vi "Read Serial Number Folder.vi"(8 "error in":errorcluster, 11 "Data IN":T1={"Message"="", "Homed?"=FALSE, "NextState"=enum."Timeout", "G.Load"=0.0, "G.Position"=0.0, "Load#"=0, "[G.Loads]"=[], "[TotalLoads]"=[], "[Errors]"=[], "ZeroWait"=0, "Results"=[], "DwellWait"=FALSE, "Test Result"=FALSE, "[CondyleLoads]"=[], "[Max]"=[], "[Min]"=[], "Valid String?"=FALSE, "ScanTime"=timestamp(0 s since 1904-01-01), "ScannedString"="", "LabelDevID"=0, "MfgDate"=timestamp(0 s since 1904-01-01), "[EEPROM Cmds]"=[], "[CalData]"=[], "[A/Ds]"=[], "[A/Dmax]"=[], "[A/Dmin]"=[], "BattMax"=0.0, "BattMin"=0.0, "DwellTime"=2000, "PendingDeviceType"="", "Zero G.load"=0.0, "GAINC Value"="", "Programming Step"=enum."Load EEPROM", "Front Panel Program?"=FALSE, "Final Program?"=FALSE, "PCB Score"=100, "AssyScore"=100, "Pass/Fail #"="", "Result String"="", "Programming Mode"=enum."Initial Program", "Angle Test Step"=enum."Initialize", "Accel Values"=[], "Shutdown Counter"=0, "V1"=0, "V2"=0, "V3"=0, "V4"=0, "EEPROM Data"=[], "Counter"=0, "Page#"=0, "Timer"=timestamp(0 s since 1904-01-01), "Use Mark10?"=FALSE, "Eng-Result#"=0, "DUT Serial #"=0, "Scroll Message?"=FALSE, "Clear Message"=FALSE, "Batt Test Step "=enum."Initialize", "RXTX Window Found?"=FALSE, "Shutdown First Call?"=FALSE, "A2 Delay (msec)"=500, "Support Script"={"Script #"="", "Script Revision"="", "[OEMs]"=[], "[[DeviceTypes]]"=[], "[[DeviceTypesVals]]"=[], "[[List of Errors]]"=[], "Default GAINC"="", "[[ASICtrims]]"=[], "ID For Echo"="", "Condyle A CalFactor"=100, "Condyle B CalFactor"=100, "[OEMs Prefix]"=[], "Packet ID 18"="", "[[Force Table Load Test]]"=[], "[[Force Table AccurTest]]"=[]}, "Serial Table"={"Serial File Path"=path "", "[[Serial Lookup Table]]"=[], "Serial Device Info"=[], "Valid Serial?"=FALSE}, "Target Information"={"Target Brand"="", "Target DeviceType"="", "Target Serial#"=100, "Target Lot#"=0, "Target DevID"=0, "Target Channel"=5}, "Operator"="", "COM Port"="", "Config Path"=path "", "Tx Array"=[], "DUT Parameters"={"Channel"=0, "DeviceID"=0, "Script Rev"=0, "Month"=0, "Day"=0, "Year"=0, "Lot#"=0, "V1"=0, "V2"=0, "V3"=0, "V4"=0, "MFG"=0, "Cal FactorA 10"=0, "Cal FactorB 10  "=0, "Cal FactorA 16"=0, "Cal FactorB 16"=0, "ASICtrim"=[], "TmpChan"=0, "GAINC"="", "Brand"="", "Device"="", "Serial #"=0, "Batt310"=0, "Batt 280"=0}, "FTS Main?"=FALSE, "Loading"={"[Forces]"=[], "[Dwell]"=[], "Loading Step"=enum."Initialize Test"}, "Software Version"="", "Correction Factor"="", "Second Load Test"=FALSE, "Acc Loads"=[], "Mark10 Config"={"H2S%"=[80.0, 85.0, 90.0, 95.0, 100.0], "H2S Speed"=[12.0, 8.0, 6.0, 4.0, 2.0], "H to S"=2.0, "Home Speed"=1.0, "LoadWin"=0.0, "Load Speed"=0.0, "PID"={"Kp"=0.04, "Kd"=0.005001, "Ki"=2.9999999999999923e-05}}, "Channels"={"Transceiver Ch"=5, "Operating Ch"=5, "Start Ch"=0}, "Channel EEPROM"=[], "Load Notes"=[], "Engr Log?"=FALSE, "Time"=[], "Program Retry"=FALSE, "Operator Channel"="", "Target Channel "="", "New Data Program"=FALSE, "NFHU Pass?"=FALSE, "Cycle Number"=0, "Cal Cycle#"=0, "[Avg G.Loads] "=[], "[Avg A/Ds] "=[], "Cal Retry?"=FALSE, "[Total A/Ds]  "=[], "Cycle Num LA"=0, "LA Cycle# "=0, "Shim Num"=0, "Shim#  "=0, "Angle Test?"=FALSE} {"Mark10 Config"."PID"."Ki" min=0.0 max=200.0 format="%.6f"; "Mark10 Config"."PID"."Kd" min=0.0 max=200.0 format="%.6f"; "Mark10 Config"."PID"."Kp" min=0.0 max=200.0 format="%.6f"; "DUT Parameters"."ASICtrim" format="%02x"}) -> (0 "error out":errorcluster, 2 "Current State Out":T2=enum."Scan Channels", 3 "State-machine Local Variables out":T1={"Message"="", "Homed?"=FALSE, "NextState"=enum."Timeout", "G.Load"=0.0, "G.Position"=0.0, "Load#"=0, "[G.Loads]"=[], "[TotalLoads]"=[], "[Errors]"=[], "ZeroWait"=0, "Results"=[], "DwellWait"=FALSE, "Test Result"=FALSE, "[CondyleLoads]"=[], "[Max]"=[], "[Min]"=[], "Valid String?"=FALSE, "ScanTime"=timestamp(0 s since 1904-01-01), "ScannedString"="", "LabelDevID"=0, "MfgDate"=timestamp(0 s since 1904-01-01), "[EEPROM Cmds]"=[], "[CalData]"=[], "[A/Ds]"=[], "[A/Dmax]"=[], "[A/Dmin]"=[], "BattMax"=0.0, "BattMin"=0.0, "DwellTime"=2000, "PendingDeviceType"="", "Zero G.load"=0.0, "GAINC Value"="", "Programming Step"=enum."Load EEPROM", "Front Panel Program?"=FALSE, "Final Program?"=FALSE, "PCB Score"=100, "AssyScore"=100, "Pass/Fail #"="", "Result String"="", "Programming Mode"=enum."Initial Program", "Angle Test Step"=enum."Initialize", "Accel Values"=[], "Shutdown Counter"=0, "V1"=0, "V2"=0, "V3"=0, "V4"=0, "EEPROM Data"=[], "Counter"=0, "Page#"=0, "Timer"=timestamp(0 s since 1904-01-01), "Use Mark10?"=FALSE, "Eng-Result#"=0, "DUT Serial #"=0, "Scroll Message?"=FALSE, "Clear Message"=FALSE, "Batt Test Step "=enum."Initialize", "RXTX Window Found?"=FALSE, "Shutdown First Call?"=FALSE, "A2 Delay (msec)"=500, "Support Script"={"Script #"="", "Script Revision"="", "[OEMs]"=[], "[[DeviceTypes]]"=[], "[[DeviceTypesVals]]"=[], "[[List of Errors]]"=[], "Default GAINC"="", "[[ASICtrims]]"=[], "ID For Echo"="", "Condyle A CalFactor"=100, "Condyle B CalFactor"=100, "[OEMs Prefix]"=[], "Packet ID 18"="", "[[Force Table Load Test]]"=[], "[[Force Table AccurTest]]"=[]}, "Serial Table"={"Serial File Path"=path "", "[[Serial Lookup Table]]"=[], "Serial Device Info"=[], "Valid Serial?"=FALSE}, "Target Information"={"Target Brand"="", "Target DeviceType"="", "Target Serial#"=100, "Target Lot#"=0, "Target DevID"=0, "Target Channel"=5}, "Operator"="", "COM Port"="", "Config Path"=path "", "Tx Array"=[], "DUT Parameters"={"Channel"=0, "DeviceID"=0, "Script Rev"=0, "Month"=0, "Day"=0, "Year"=0, "Lot#"=0, "V1"=0, "V2"=0, "V3"=0, "V4"=0, "MFG"=0, "Cal FactorA 10"=0, "Cal FactorB 10  "=0, "Cal FactorA 16"=0, "Cal FactorB 16"=0, "ASICtrim"=[], "TmpChan"=0, "GAINC"="", "Brand"="", "Device"="", "Serial #"=0, "Batt310"=0, "Batt 280"=0}, "FTS Main?"=FALSE, "Loading"={"[Forces]"=[], "[Dwell]"=[], "Loading Step"=enum."Initialize Test"}, "Software Version"="", "Correction Factor"="", "Second Load Test"=FALSE, "Acc Loads"=[], "Mark10 Config"={"H2S%"=[80.0, 85.0, 90.0, 95.0, 100.0], "H2S Speed"=[12.0, 8.0, 6.0, 4.0, 2.0], "H to S"=2.0, "Home Speed"=1.0, "LoadWin"=0.0, "Load Speed"=0.0, "PID"={"Kp"=0.04, "Kd"=0.005001, "Ki"=2.9999999999999923e-05}}, "Channels"={"Transceiver Ch"=5, "Operating Ch"=5, "Start Ch"=0}, "Channel EEPROM"=[], "Load Notes"=[], "Engr Log?"=FALSE, "Time"=[], "Program Retry"=FALSE, "Operator Channel"="", "Target Channel "="", "New Data Program"=FALSE, "NFHU Pass?"=FALSE, "Cycle Number"=0, "Cal Cycle#"=0, "[Avg G.Loads] "=[], "[Avg A/Ds] "=[], "Cal Retry?"=FALSE, "[Total A/Ds]  "=[], "Cycle Num LA"=0, "LA Cycle# "=0, "Shim Num"=0, "Shim#  "=0, "Angle Test?"=FALSE} {"Mark10 Config"."PID"."Ki" min=0.0 max=200.0 format="%.6f"; "Mark10 Config"."PID"."Kd" min=0.0 max=200.0 format="%.6f"; "Mark10 Config"."PID"."Kp" min=0.0 max=200.0 format="%.6f"; "DUT Parameters"."ASICtrim" format="%02x"})   [LabVIEW 2015]
uses:
  Controls/LocalVars.ctl
  Controls/Gen2 FT states.ctl
  Controls/Iniial Device Programming.ctl
  ProgramStageControl.ctl
  Controls/Batt Cap Steps.ctl
  Controls/Support Script.ctl
  Controls/Serial Table.ctl
  Controls/Device Information.ctl
  Controls/InfoPacket.ctl
  Controls/Loading.ctl
  Controls/Load Step.ctl
  Controls/Mark10 Config.ctl
  Controls/PID parameters.ctl
  Controls/Channels.ctl
  <vilib>/Utility/config.llb/Write Key (Path).vi
  <vilib>/Utility/config.llb/NI_LVConfig.lvlib
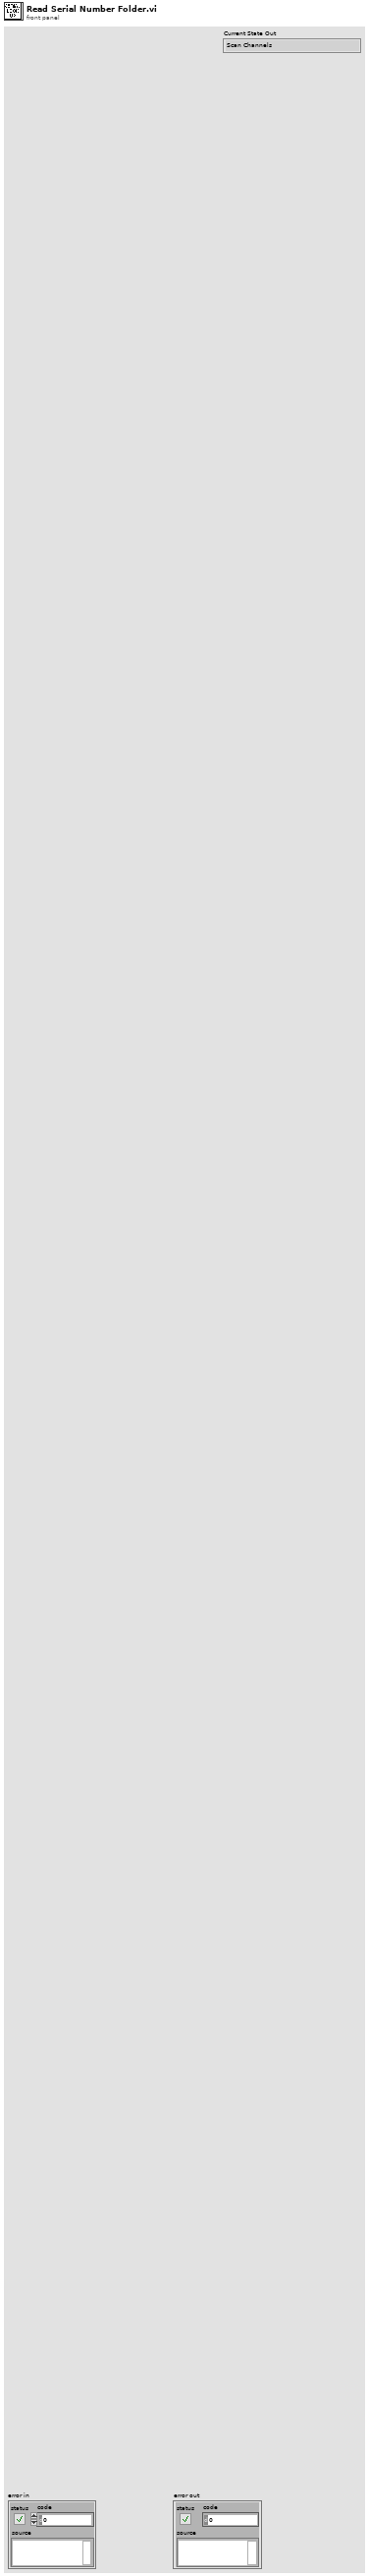
[diagram p1: front panel]
types:
  T1 = typedef "LocalVars.ctl" = cluster{"Message":string, "Homed?":bool, "NextState":T2, "G.Load":dbl, "G.Position":dbl, "Load#":i32, "[G.Loads]":dbl[], "[TotalLoads]":dbl[], "[Errors]":dbl[][], "ZeroWait":u32, "Results":dbl[], "DwellWait":bool, "Test Result":bool, "[CondyleLoads]":dbl[][], "[Max]":dbl[], "[Min]":dbl[], "Valid String?":bool, "ScanTime":timestamp, "ScannedString":string, "LabelDevID":u32, "MfgDate":timestamp, "[EEPROM Cmds]":u8[][], "[CalData]":u8[][], "[A/Ds]":dbl[][], "[A/Dmax]":dbl[], "[A/Dmin]":dbl[], "BattMax":dbl, "BattMin":dbl, "DwellTime":i32, "PendingDeviceType":string, "Zero G.load":dbl, "GAINC Value":string, "Programming Step":T3, "Front Panel Program?":bool, "Final Program?":bool, "PCB Score":i32, "AssyScore":i32, "Pass/Fail #":string, "Result String":string, "Programming Mode":T4, "Angle Test Step":enum16{"Initialize", "Get X", "Get Y", "Get Z", "Next Test"}, "Accel Values":dbl[][], "Shutdown Counter":u32, "V1":i32, "V2":i32, "V3":i32, "V4":i32, "EEPROM Data":i32[][], "Counter":i32, "Page#":i32, "Timer":timestamp, "Use Mark10?":bool, "Eng-Result#":u32, "DUT Serial #":i32, "Scroll Message?":bool, "Clear Message":bool, "Batt Test Step ":T5, "RXTX Window Found?":bool, "Shutdown First Call?":bool, "A2 Delay (msec)":i16, "Support Script":T6, "Serial Table":T7, "Target Information":T8, "Operator":string, "COM Port":string, "Config Path":path, "Tx Array":u8[], "DUT Parameters":T9, "FTS Main?":bool, "Loading":T10, "Software Version":string, "Correction Factor":string, "Second Load Test":bool, "Acc Loads":dbl[][], "Mark10 Config":T12, "Channels":T14, "Channel EEPROM":i32[][], "Load Notes":string[], "Engr Log?":bool, "Time":timestamp[], "Program Retry":bool, "Operator Channel":string, "Target Channel ":string, "New Data Program":bool, "NFHU Pass?":bool, "Cycle Number":i32, "Cal Cycle#":i32, "[Avg G.Loads] ":dbl[], "[Avg A/Ds] ":dbl[][], "Cal Retry?":bool, "[Total A/Ds]  ":dbl[][], "Cycle Num LA":i32, "LA Cycle# ":i32, "Shim Num":i32, "Shim#  ":i32, "Angle Test?":bool}
  T2 = typedef "Gen2 FT states.ctl" = enum16{"---------SETUP-------", "Initialization", "Read Support Data", "Initialize Mark-10", "Initialize Transceiver", "------UTILITIES------", "Change DUT Channel", "Find RxTx Window", "Reset Device", "Scan Channels", "Read Serial Lookup", "Shutdown Device", "ESTOP", "--------USER---------", "Timeout", "-----PROGRAM-----", "Program Device", "------MARK10--------", "Go Home", "MoveUp", "MoveDown", "Goto Load", "Goto Position", "Stop Motor", "---------TESTS--------", "Start Test", "Angle Test", "Load Test", "Load Accuracy Test", "Battery Test", "------RESULTS-------", "End Test", "Display Result", "--------EXIT--------", "Exit"}
  T3 = typedef "Iniial Device Programming.ctl" = enum16{"Load EEPROM", "Send First A1", "Send EEPROM", "Send A1", "Check EEPROM Echo", "Verify transmission", "Programming Successful", "Programming Failed"}
  T4 = typedef "ProgramStageControl.ctl" = enum16{"Initial Program", "GainC", "Scales"}
  T5 = typedef "Batt Cap Steps.ctl" = enum16{"Initialize", "Collect 2.8 Volts", "Collect 3.1 Volts", "Check Results"}
  T6 = typedef "Support Script.ctl" = cluster{"Script #":string, "Script Revision":string, "[OEMs]":string[], "[[DeviceTypes]]":string[][], "[[DeviceTypesVals]]":u16[][], "[[List of Errors]]":string[][], "Default GAINC":string, "[[ASICtrims]]":u8[][], "ID For Echo":string, "Condyle A CalFactor":i32, "Condyle B CalFactor":i32, "[OEMs Prefix]":string[], "Packet ID 18":string, "[[Force Table Load Test]]":dbl[][], "[[Force Table AccurTest]]":dbl[][]}
  T7 = typedef "Serial Table.ctl" = cluster{"Serial File Path":path, "[[Serial Lookup Table]]":string[][], "Serial Device Info":string[], "Valid Serial?":bool}
  T8 = typedef "Device Information.ctl" = cluster{"Target Brand":string, "Target DeviceType":string, "Target Serial#":i32, "Target Lot#":u32, "Target DevID":u32, "Target Channel":u8}
  T9 = typedef "InfoPacket.ctl" = cluster{"Channel":u8, "DeviceID":u32, "Script Rev":u8, "Month":u8, "Day":u8, "Year":u8, "Lot#":u32, "V1":u16, "V2":u16, "V3":u16, "V4":u16, "MFG":u8, "Cal FactorA 10":u8, "Cal FactorB 10  ":u8, "Cal FactorA 16":u8, "Cal FactorB 16":u8, "ASICtrim":u8[], "TmpChan":u8, "GAINC":string, "Brand":string, "Device":string, "Serial #":u64, "Batt310":u16, "Batt 280":u16}
  T10 = typedef "Loading.ctl" = cluster{"[Forces]":dbl[], "[Dwell]":dbl[], "Loading Step":T11}
  T11 = typedef "Load Step.ctl" = enum16{"Initialize Test", "Go Home", "Detect Dev Surface", "Wait to zero Device", "Zero Device", "Do Test", "Test Result"}
  T12 = typedef "Mark10 Config.ctl" = cluster{"H2S%":dbl[], "H2S Speed":dbl[], "H to S":dbl, "Home Speed":dbl, "LoadWin":dbl, "Load Speed":dbl, "PID":T13}
  T13 = typedef "PID parameters.ctl" = cluster{"Kp":dbl, "Kd":dbl, "Ki":dbl}
  T14 = typedef "Channels.ctl" = cluster{"Transceiver Ch":u8, "Operating Ch":u8, "Start Ch":u8}
  T15 = typedef "NI_LVConfig.lvlib/Config Data RefNum.ctl" = refnum<k1>
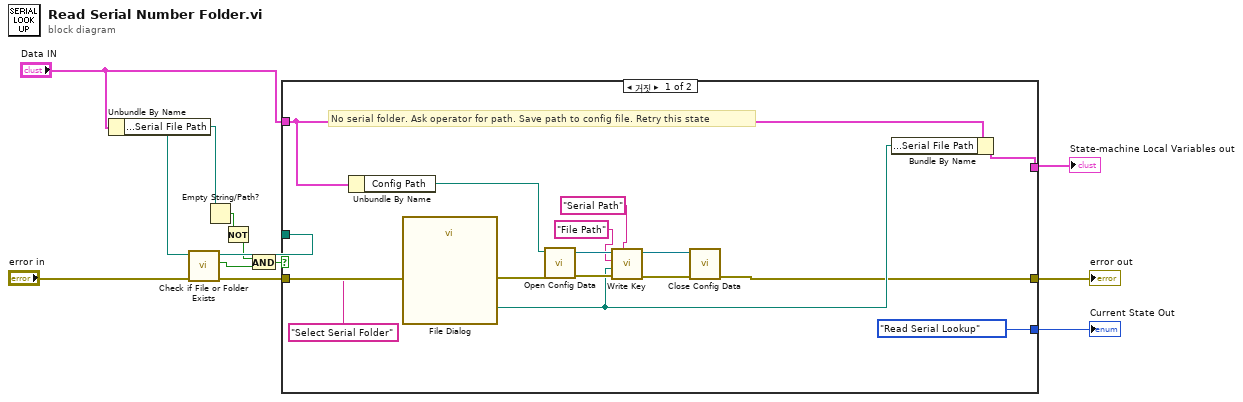
[diagram p0: block diagram]
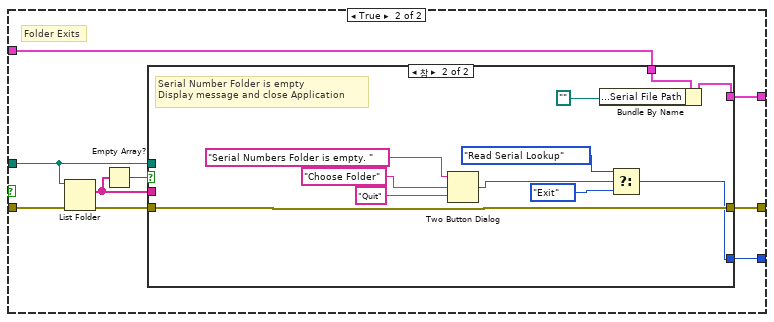
[diagram p2: hidden frame]
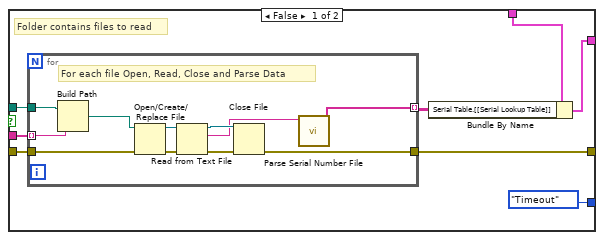
[diagram p3: hidden frame]
diagram:
  n1 = Unbundle By Name("Data IN") -> ("Serial Table.Serial File Path"=w5:path)
  n2 = call <vilib>:"Check if File or Folder Exists.vi"("error in (no error)"="error in", "path"=w5) -> ("error out"=w7:errorcluster, "file or folder exists?"=w3:bool, "dup path"=w6:path)  [unwired: 7 in]
  n3 = Empty String/Path?(string/path=w5) -> (empty?=w4:bool)
  n4 = Not(x=w4) -> (.not. x?=w1:bool)
  n5 = And(x=w1, y=w3) -> (x .and. y?=w2:bool)
  n6 = case shown="거짓" w2 {
    tunnel: [Gen2_FT_states."Read Serial Lookup" ("Current State Out") w32] -> w10
    tunnel: w7 -> [w25 w36]
    tunnel: [w15 w33] -> w11
    tunnel: w6 -> [_ w30]
    tunnel: "Data IN" -> [w24 w29]
    tunnel: [w26 w28] -> w12
    frame False {
      # "No serial folder. Ask operator for path. Save path to config file. Retry this state"
      n7 = Unbundle By Name(w24) -> ("Config Path"=w22:path)
      n8 = call "File Dialog"("prompt"="Select Serial Folder", "error in"=w25) -> ("selected path"=w17:path, "error out"=w23:errorcluster)  [unwired: 10 in, 2 out]
      n9 = call <vilib>:"Open Config Data.vi"("error in (no error)"=w23, "configuration file path"=w22) -> ("error out"=w21:errorcluster, "refnum"=w20:T15)  [unwired: 7 in, 1 out]
      n10 = call-poly <vilib>:"Write Key.vi"("section"="Serial Path", "error in (no error)"=w21, "value"=w17, "key"="File Path", "refnum"=w20) -> ("error out"=w16:errorcluster, "refnum out"=w14:T15)  [unwired: 4 in, 1 out]
      n11 = call <vilib>:"Close Config Data.vi"("error in (no error)"=w16, "refnum"=w14) -> ("error out"=w15:errorcluster)  [unwired: 8 in, 1 out]
      n12 = Bundle By Name(cluster=w24, "Serial Table.Serial File Path"=w17) -> (w26:T1)
    }
    frame True {
      # "Folder Exits"
      n13 = List Folder(path=w30, error in=w36) -> (filenames=w31:string[], error out=w34:errorcluster)  [unwired: 2 in, 2 out]
      n14 = Empty Array?(array=w31) -> (empty?=w35:bool)
      n15 = case shown="참" w35 {
        tunnel: w34 -> [w42 w66]
        tunnel: [w41 w66] -> w33
        tunnel: [Gen2_FT_states."Timeout" ("Current State Out") w57] -> w32
        tunnel: w31 -> [w44 _]
        tunnel: w30 -> [w43 _]
        tunnel: w29 -> [w40 w64]
        tunnel: [w39 w63] -> w28
        frame False {
          # "Folder contains files to read"
          n16 = for {
            tunnel: w44 -> [w54] mode=indexing
            tunnel: w43 -> [w55]
            tunnel: w42 -> [w53]
            tunnel: [w48] -> w41
            tunnel: [w45] -> w38 mode=indexing
            # "For each file Open, Read, Close and Parse Data"
            n17 = Build Path(base path=w55, name or relative path=w54) -> (appended path=w52:path)
            n18 = Open/Create/Replace File(file path (use dialog)=w52, error in=w53) -> (refnum out=w50:refnum<file>, error out=w51:errorcluster)  [unwired: 4 in, 1 out]
            n19 = Read from Text File(file (use dialog)=w50, error in=w51) -> (refnum out=w47:refnum<file>, text=w46:string, error out=w49:errorcluster)  [unwired: 2 in, 1 out]
            n20 = Close File(refnum=w47, error in=w49) -> (error out=w48:errorcluster)  [unwired: 1 out]
            n21 = call "Parse Serial Number File.vi"("String"=w46) -> ("Array"=w45:string[])  [unwired: 10 in]
          }
          n22 = Bundle By Name(cluster=w40, "Serial Table.[[Serial Lookup Table]]"=w38) -> (w39:T1)
        }
        frame True {
          # "Serial Number Folder is empty\nDisplay message and close Application"
          n23 = Two Button Dialog(message="Serial Numbers Folder is empty. ", 1:"Quit" ("F button name (\"Cancel\")"), 2:"Choose Folder" ("T button name (\"OK\")")) -> (T button?=w59:bool)
          n24 = Bundle By Name(cluster=w64, "Serial Table.Serial File Path"=path "") -> (w63:T1)
          n25 = Select(t=Gen2_FT_states."Read Serial Lookup" ("Current State Out"), s=w59, f=Gen2_FT_states."Exit") -> (s? t:f=w57:T2)
        }
      }
    }
  }
  "State-machine Local Variables out" <- w12
  "error out" <- w11
  "Current State Out" <- w10
